vi "Write password.vi"(8 "error in (no error)":errorcluster, 10 "password":string, 11 "OpenSSH Client in":refnum<class "OpenSSH Client.lvclass">) -> (0 "error out":errorcluster, 3 "OpenSSH Client out":refnum<class "OpenSSH Client.lvclass">)   [LabVIEW 2020, in "NI_SSH.lvlib" / "OpenSSH Client.lvclass"]
uses:
  <vilib>/net/SSH/Client/OpenSSH/OpenSSH Client.lvclass
  <vilib>/Utility/error.llb/Error Cluster From Error Code.vi
  <vilib>/ErrorRing/Error Ring.xnode
  <vilib>/net/SSH/Client/Generic/Generic Client.lvclass
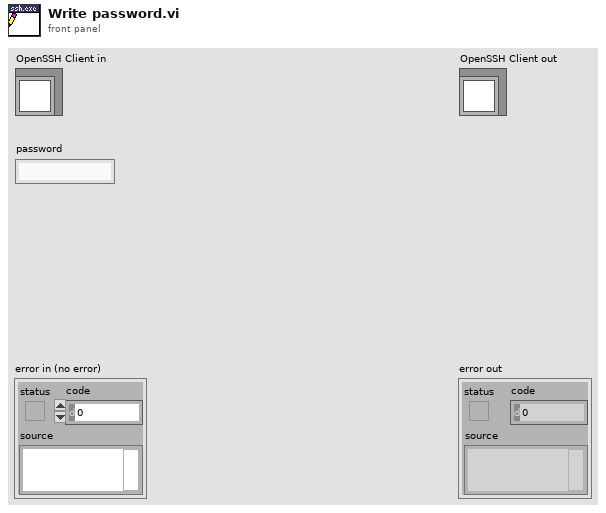
[diagram p1: front panel]
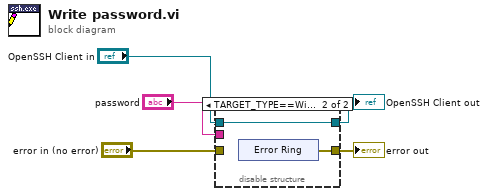
[diagram p0: block diagram]
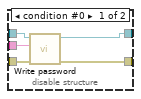
[diagram p2: hidden frame]
diagram:
  n1 = disable-structure "Conditional Disable Structure" shown="TARGET_TYPE==Windows||OS==Win" {
    disable-tunnel: [w10 w12] -> w5
    disable-tunnel: [w9 w11] -> w4
    disable-tunnel: "error in (no error)" -> [w8 _]
    disable-tunnel: "password" -> [w7 _]
    disable-tunnel: "OpenSSH Client in" -> [w6 w11]
    frame condition #0 {
      n2 = call-parent "Write password.vi"("error in (no error)"=w8, "password"=w7, "Generic Client in"=w6) -> ("error out"=w10:errorcluster, "Generic Client out"=w9:refnum<class "OpenSSH Client.lvclass">)  [unwired: 7 in]
    }
    frame condition #1 (active) {
      n3 = xnode ("Error Ring")() -> ("error out"=w12:errorcluster)
    }
  }
  "error out" <- w5
  "OpenSSH Client out" <- w4
